vi "Termopar.vi"() -> ()   [LabVIEW 2014]
panel:
  out "Temperature (degC)":dbl
  out "Input Voltage (mV)":dbl
  out "Emf(Thermocouple - mV)":dbl
  out "Emf(Hot-mV)":dbl
  in  "Thermocouple (degC)":dbl min=0.0 max=1000.0 step=1.0
  out "LM35 temperature (degC)":dbl
  in  "stop":bool
  out "Emf(Cold - mV)":dbl
  in  "LM35 output (mv)":dbl min=0.0 max=100.0 step=0.01
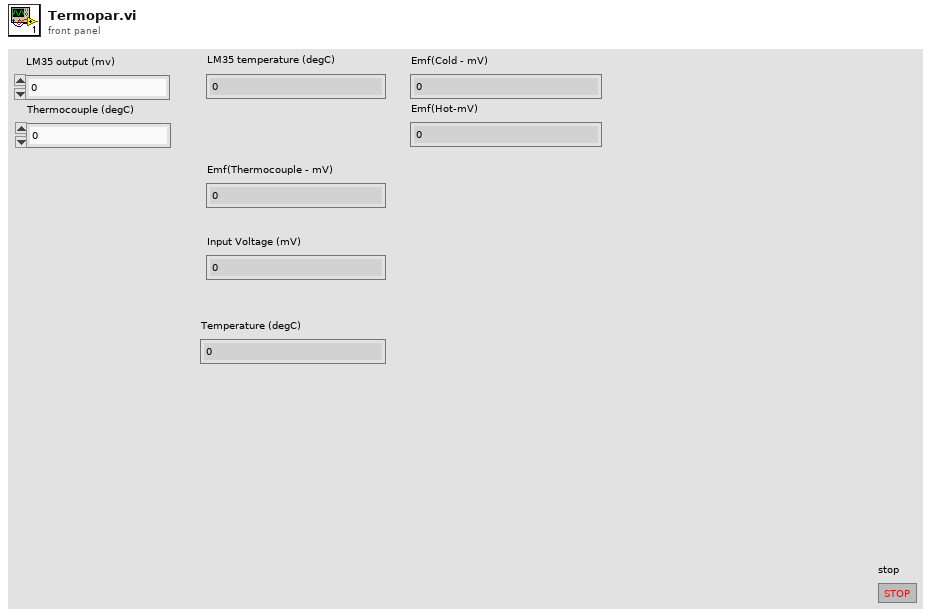
[diagram p1: front panel]
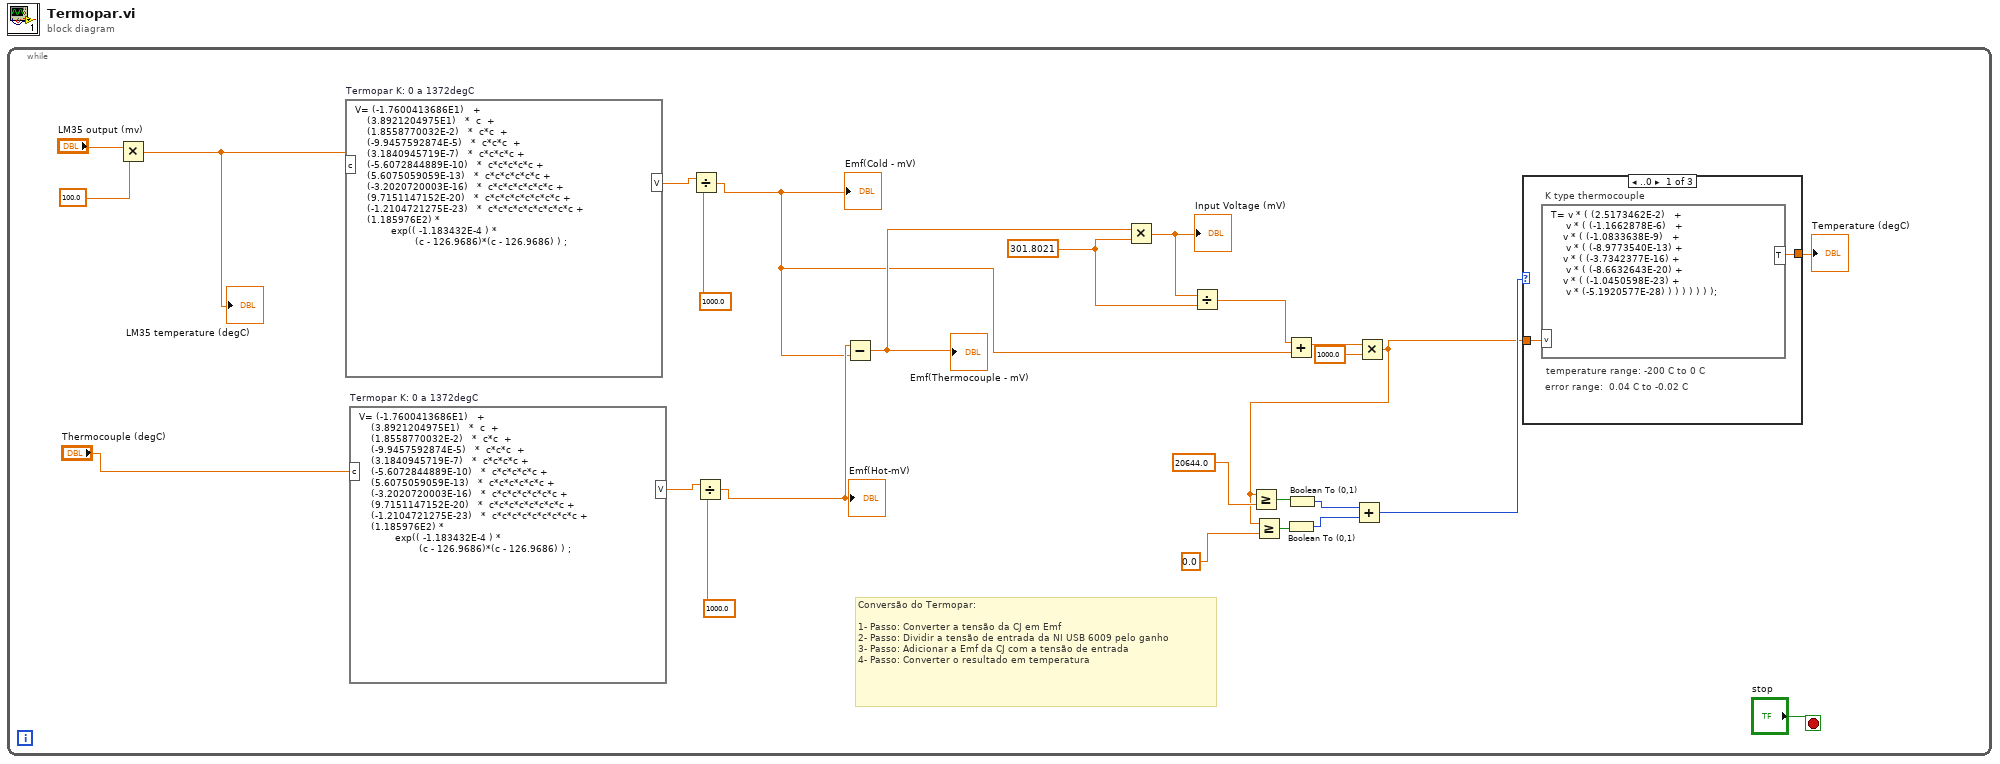
[diagram p0: block diagram]
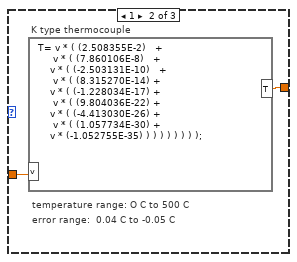
[diagram p2: hidden frame]
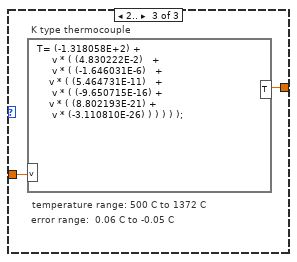
[diagram p3: hidden frame]
diagram:
  n1 = while {
    stop <- "stop" stop-if-true
    w14 = 301.8021 ("y")
    # "Conversão do Termopar:\n\n1- Passo: Converter a tensão da CJ em Emf\n2- Passo: Dividir a tensão de entrada da NI USB 6009 pelo ganho\n3- Passo: Adicionar a Emf da CJ com a tensão de entrada\n4- Passo: Converter o resultado em temperatura"
    n2 = Multiply(x="LM35 output (mv)", y=100.0) -> (x*y=w21:dbl)
    "LM35 temperature (degC)" <- w21
    n3 = formula code="V= (-1.7600413686E1)   +\n    (3.8921204975E1)   *  c  +\n    (1.8558770032E-2)   *  c*c  +\n    (-9.9457592874E-5)   *  c*c*c  +\n    (3.1840945719E-7)   *  c*c*c*c +\n    (-5.6072844889E-10)   *  c*c*c*c*c +\n    (5.6075059059E-13)   *  c*c*c*c*c*c +\n    (-3.2020720003E-16)   *  c*c*c*c*c*c*c +\n    (9.7151147152E-20)   *  c*c*c*c*c*c*c*c +\n    (-1.2104721275E-23)   *  c*c*c*c*c*c*c*c*c +\n    (1.185976E2) * \n            exp(( -1.183432E-4 ) * \n                    (c - 126.9686)*(c - 126.9686) ) ;" "Termopar K: 0 a 1372degC"("c"=w21) -> ("V"=w24:dbl)
    n4 = formula code="V= (-1.7600413686E1)   +\n    (3.8921204975E1)   *  c  +\n    (1.8558770032E-2)   *  c*c  +\n    (-9.9457592874E-5)   *  c*c*c  +\n    (3.1840945719E-7)   *  c*c*c*c +\n    (-5.6072844889E-10)   *  c*c*c*c*c +\n    (5.6075059059E-13)   *  c*c*c*c*c*c +\n    (-3.2020720003E-16)   *  c*c*c*c*c*c*c +\n    (9.7151147152E-20)   *  c*c*c*c*c*c*c*c +\n    (-1.2104721275E-23)   *  c*c*c*c*c*c*c*c*c +\n    (1.185976E2) * \n            exp(( -1.183432E-4 ) * \n                    (c - 126.9686)*(c - 126.9686) ) ;" "Termopar K: 0 a 1372degC"("c"="Thermocouple (degC)") -> ("V"=w20:dbl)
    n5 = Divide(x=w24, y=1000.0) -> (x/y=w12:dbl)
    "Emf(Cold - mV)" <- w12
    n6 = Divide(x=w20, y=1000.0) -> (x/y=w16:dbl)
    "Emf(Hot-mV)" <- w16
    n7 = Subtract(x=w16, y=w12) -> (x-y=w17:dbl)
    "Emf(Thermocouple - mV)" <- w17
    n8 = Multiply(x=w17, y=w14) -> (x*y=w15:dbl)
    "Input Voltage (mV)" <- w15
    n9 = Divide(x=w15, y=w14) -> (x/y=w13:dbl)
    n10 = Add(x=w13, y=w12) -> (x+y=w3:dbl)
    n11 = Multiply(x=w3, y=1000.0) -> (x*y=w1:dbl)
    n12 = Greater Or Equal?(x=w1, y=20644.0) -> (x >= y?=w9:bool)
    n13 = Greater Or Equal?(x=w1, y=0.0) -> (x >= y?=w8:bool)
    n14 = Boolean To (0,1)(Boolean=w8) -> (0, 1=w10:i16)
    n15 = Boolean To (0,1)(Boolean=w9) -> (0, 1=w11:i16)
    n16 = Add(x=w11, y=w10) -> (x+y=w5:i16)
    n17 = case shown="..0" w5 {
      tunnel: w1 -> [w27 w29 w32]
      tunnel: [w28 w30 w31] -> w4
      frame ..0 {
        # "error range:  0.04 C to -0.02 C"
        # "temperature range: -200 C to 0 C"
        # "K type thermocouple"
        n18 = formula code="T= v * ( (2.5173462E-2)   +\n     v * ( (-1.1662878E-6)   +\n    v * ( (-1.0833638E-9)   +\n     v * ( (-8.9773540E-13) +\n    v * ( (-3.7342377E-16) +\n     v * ( (-8.6632643E-20) +\n    v * ( (-1.0450598E-23) +\n     v * (-5.1920577E-28) ) ) ) ) ) ) );"("v"=w27) -> ("T"=w28:dbl)
      }
      frame 1 {
        # "error range:  0.04 C to -0.05 C"
        # "temperature range: O C to 500 C"
        # "K type thermocouple"
        n19 = formula code="T= v * ( (2.508355E-2)   +\n     v * ( (7.860106E-8)   +\n    v * ( (-2.503131E-10)   +\n     v * ( (8.315270E-14) +\n    v * ( (-1.228034E-17) +\n     v * ( (9.804036E-22) +\n    v * ( (-4.413030E-26) +\n     v * ( (1.057734E-30) +               \n    v * (-1.052755E-35) ) ) ) ) ) ) ) );"("v"=w29) -> ("T"=w30:dbl)
      }
      frame 2.. {
        # "error range:  0.06 C to -0.05 C"
        # "temperature range: 500 C to 1372 C"
        # "K type thermocouple"
        n20 = formula code="T= (-1.318058E+2) +\n     v * ( (4.830222E-2)   +\n     v * ( (-1.646031E-6)   +\n    v * ( (5.464731E-11)   +\n     v * ( (-9.650715E-16) +\n    v * ( (8.802193E-21) +\n     v * (-3.110810E-26) ) ) ) ) );"("v"=w32) -> ("T"=w31:dbl)
      }
    }
    "Temperature (degC)" <- w4
  }
